vi "Infer top player action indicators.vi"(1 "Movement data with player transitions notated":string[][](array[string])=array1935x4[7740 elements]) -> (0 "Top player infered actions column":string[](array[string]))   [LabVIEW 2014]
panel:
  out "Top player action notated":string[][](array[string])
  out "Array 5":i32[][](array[numeric])
  out "Array":i32[][](array[numeric])
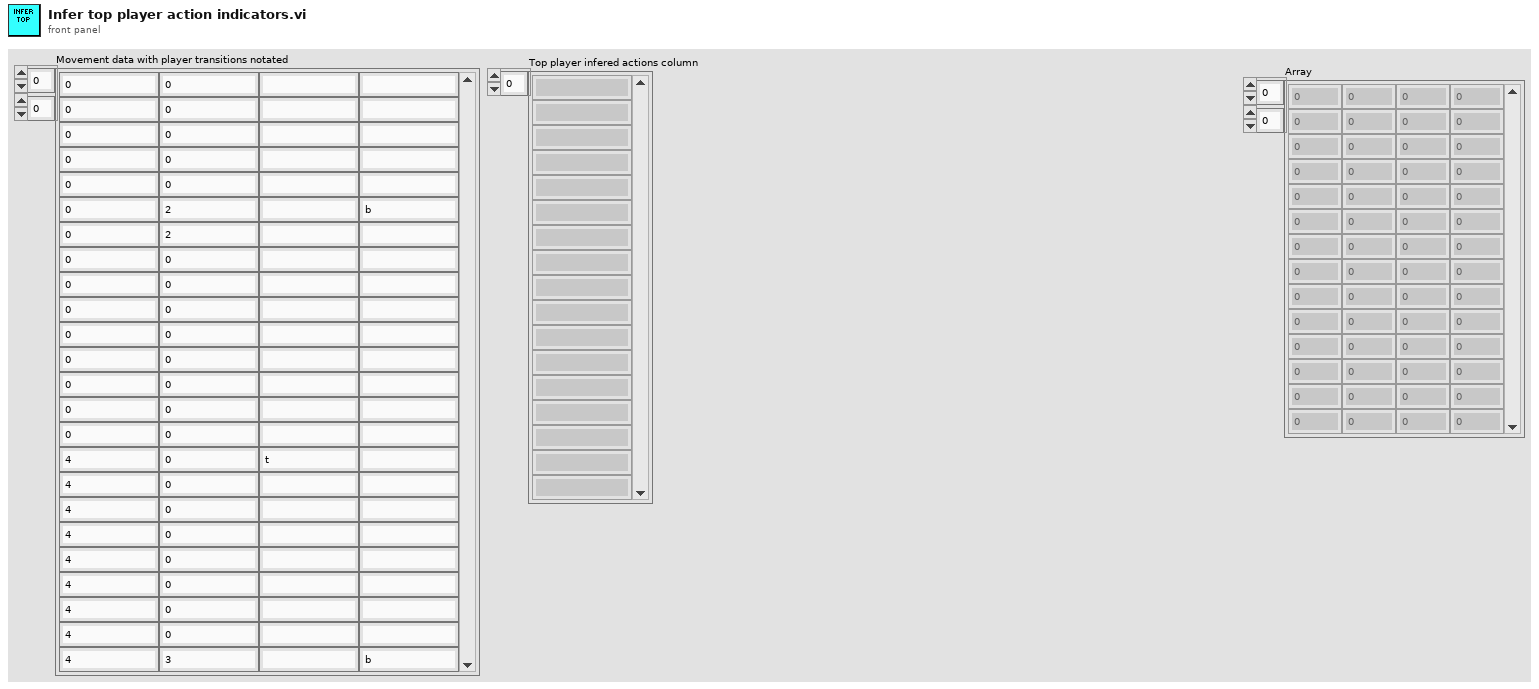
[diagram p1: front panel]
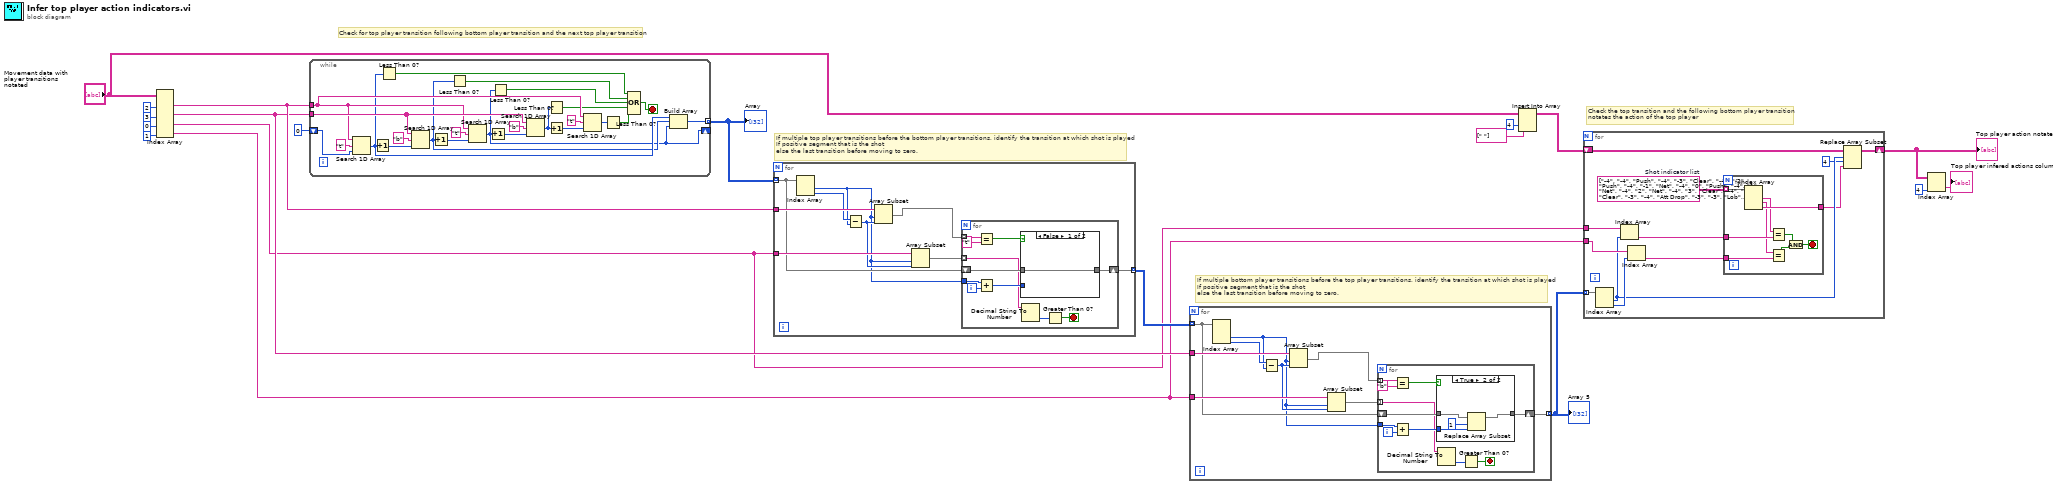
[diagram p0: block diagram]
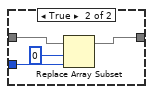
[diagram p3: hidden frame]
diagram:
  # "Check the top transition and the following bottom player transition\nnotates the action of the top player"
  # "If multiple bottom player transitions before the top player transitions, identify the transition at which shot is played\nIf positive segment that is the shot\nelse the last transition before moving to zero."
  # "If multiple top player transitions before the bottom player transitions, identify the transition at which shot is played\nIf positive segment that is the shot\nelse the last transition before moving to zero."
  # "Check for top player transition following bottom player transition and the next top player transition"
  n1 = Index Array(array="Movement data with player transitions notated", index (col) #1=2 ("disabled index (col)"), index (col) #2=3 ("index (col)"), index (col) #3=0 ("index (col)"), index (col) #4=1 ("index (col)")) -> (element #1=w16:string[], element #2=w12:string[], element #3=w8:string[], element #4=w9:string[])  [unwired: 4 in]
  n2 = while {
    tunnel: w16 -> [w33]
    tunnel: w12 -> [w34]
    shift-right: [w23] -> _
    shift-left: 0 ("index (col)") -> [w42]
    tunnel: [w39] -> w13 mode=indexing
    stop <- w26 stop-if-true
    n3 = Search 1D Array(1D array=w33, element="t", start index (0)=w42) -> (index of element=w25:i32)
    n4 = Increment(x=w25) -> (x+1=w38:i32)
    n5 = Less Than 0?(x=w25) -> (x < 0?=w22:bool)
    n6 = Search 1D Array(1D array=w34, element="b", start index (0)=w38) -> (index of element=w24:i32)
    n7 = Increment(x=w24) -> (x+1=w37:i32)
    n8 = Less Than 0?(x=w24) -> (x < 0?=w21:bool)
    n9 = Search 1D Array(1D array=w33, element="t", start index (0)=w37) -> (index of element=w23:i32)
    n10 = Increment(x=w23) -> (x+1=w35:i32)
    n11 = Less Than 0?(x=w23) -> (x < 0?=w20:bool)
    n12 = Search 1D Array(1D array=w34, element="b", start index (0)=w35) -> (index of element=w30:i32)
    n13 = Less Than 0?(x=w30) -> (x < 0?=w28:bool)
    n14 = Increment(x=w30) -> (x+1=w31:i32)
    n15 = Search 1D Array(1D array=w33, element="t", start index (0)=w31) -> (index of element=w29:i32)
    n16 = Less Than 0?(x=w29) -> (x < 0?=w27:bool)
    n17 = Compound Arithmetic op=OR(w22, w21, w20, w28, w27) -> (w26:bool)
    n18 = Build Array(w25, w24, w23) -> (w39:i32[])
  }
  "Array" <- w13
  n19 = for {
    tunnel: w13 -> [w46] mode=indexing
    tunnel: w16 -> [w52]
    tunnel: w8 -> [w50]
    tunnel: [w45] -> w11 mode=indexing
    n20 = Index Array(array=w46) -> (element #1=w44:i32, element #2=w51:i32)  [unwired: 2 in]
    n21 = Subtract(x=w51, y=w44) -> (x-y=w49:i32)
    n22 = Array Subset(array=w52, index=w44, length=w49) -> (w48:string[])
    n23 = Array Subset(array=w50, index=w44, length=w49) -> (w47:string[])
    n24 = for {
      tunnel: w48 -> [w63] mode=indexing
      tunnel: w47 -> [w56] mode=indexing
      tunnel: w44 -> [w60]
      shift-right: [w57] -> w45
      shift-left: w46 -> [w59]
      i -> [w61]
      stop <- w53 stop-if-true
      n25 = Equal?(x=w63, y="t") -> (x = y?=w55:bool)
      n26 = Add(x=w60, y=w61) -> (x+y=w58:i32)
      n27 = case shown="False" w55 {
        tunnel: w59 -> [w64 w68]
        tunnel: w58 -> [_ w67]
        tunnel: [w64 w65] -> w57
        frame False {
        }
        frame True {
          n28 = Replace Array Subset(array=w68, new element=w67, index=0) -> (w65:i32[])
        }
      }
      n29 = Decimal String To Number(string=w56) -> (number=w54:i32)  [unwired: 2 in, 1 out]
      n30 = Greater Than 0?(x=w54) -> (x > 0?=w53:bool)
    }
  }
  n31 = for {
    tunnel: w11 -> [w72] mode=indexing
    tunnel: w12 -> [w77]
    tunnel: w9 -> [w76]
    tunnel: [w71] -> w10 mode=indexing
    n32 = Index Array(array=w72) -> (element #2=w69:i32, element #3=w70:i32)  [unwired: 3 in, 1 out]
    n33 = Subtract(x=w70, y=w69) -> (x-y=w75:i32)
    n34 = Array Subset(array=w77, index=w69, length=w75) -> (w74:string[])
    n35 = Array Subset(array=w76, index=w69, length=w75) -> (w73:string[])
    n36 = for {
      tunnel: w74 -> [w88] mode=indexing
      tunnel: w73 -> [w81] mode=indexing
      tunnel: w69 -> [w85]
      shift-right: [w82] -> w71
      shift-left: w72 -> [w84]
      i -> [w86]
      stop <- w78 stop-if-true
      n37 = Equal?(x=w88, y="b") -> (x = y?=w80:bool)
      n38 = Add(x=w85, y=w86) -> (x+y=w83:i32)
      n39 = case shown="True" w80 {
        tunnel: w84 -> [w89 w93]
        tunnel: w83 -> [_ w92]
        tunnel: [w89 w90] -> w82
        frame False {
        }
        frame True {
          n40 = Replace Array Subset(array=w93, new element=w92, index=1) -> (w90:i32[])
        }
      }
      n41 = Decimal String To Number(string=w81) -> (number=w79:i32)  [unwired: 2 in, 1 out]
      n42 = Greater Than 0?(x=w79) -> (x > 0?=w78:bool)
    }
  }
  "Array 5" <- w10
  n43 = Insert Into Array(array="Movement data with player transitions notated", index (col)=4 ("disabled index (col)"), new element=string[] [" "] ("new element/subarray")) -> (w5:string[][])  [unwired: 1 in]
  n44 = for {
    tunnel: w10 -> [w105] mode=indexing
    tunnel: w9 -> [w103]
    tunnel: w8 -> [w104]
    shift-right: [w94] -> w3
    shift-left: w5 -> [w98]
    w101 = string[][] [["-4", "-4", "Push"], ["-4", "-3", "Clear"], ["-4", "-2", "Push"], ["-4", "-1", "Net"], ["-4", "0", "Push"], ["-4", "1", "Net"], ["-4", "2", "Net"], ["-4", "3", "Clear"], ["-4", "4", "Clear"], ["-3", "-4", "Att Drop"], ["-3", "-3", "Lob"], ["-3", "-2", "Att Drop"], ["-3", "-1", "Def Drop"], ["-3", "0", "Att Drop"], ["-3", "1", "Def Drop"], ["-3", "2", "Def Drop"], ["-3", "3", "Lob"], ["-3", "4", "Lob"], ["-2", "-4", "Push"], ["-2", "-3", "Clear"], ["-2", "-2", "Push"], ["-2", "-1", "Net"], ["-2", "0", "Push"], ["-2", "1", "Net"], ["-2", "2", "Net"], ["-2", "3", "Clear"], ["-2", "4", "Clear"], ["-1", "-4", "Deep Net"], ["-1", "-3", "Clear"], ["-1", "-2", "Deep Net"], ["-1", "-1", "Net"], ["-1", "0", "Deep Net"], ["-1", "1", "Net"], ["-1", "2", "Net"], ["-1", "3", "Clear"], ["-1", "4", "Clear"], ["0", "-4", "Push"], ["0", "-3", "Clear"], ["0", "-2", "Push"], ["0", "-1", "Net"], ["0", "0", "Push"], ["0", "1", "Net"], ["0", "2", "Net"], ["0", "3", "Clear"], ["0", "4", "Clear"], ["1", "-4", "Deep Net"], ["1", "-3", "Clear"], ["1", "-2", "Deep Net"], ["1", "-1", "Net"], ["1", "0", "Deep Net"], ["1", "1", "Net"], ["1", "2", "Net"], ["1", "3", "Clear"], ["1", "4", "Clear"], ["2", "-4", "Deep Net"], ["2", "-3", "Clear"], ["2", "-2", "Deep Net"], ["2", "-1", "Net"], ["2", "0", "Deep Net"], ["2", "1", "Net"], ["2", "2", "Net"], ["2", "3", "Clear"], ["2", "4", "Clear"], ["3", "-4", "Att Drop"], ["3", "-3", "Lob"], ["3", "-2", "Att Drop"], ["3", "-1", "Def Drop"], ["3", "0", "Att Drop"], ["3", "1", "Def Drop"], ["3", "2", "Def Drop"], ["3", "3", "Lob"], ["3", "4", "Lob"], ["4", "-4", "Att Drop"], ["4", "-3", "Lob"], ["4", "-2", "Att Drop"], ["4", "-1", "Def Drop"], ["4", "0", "Att Drop"], ["4", "1", "Def Drop"], ["4", "2", "Def Drop"], ["4", "3", "Lob"], ["4", "4", "Lob"]]  # Shot indicator list
    n45 = Index Array(array=w105) -> (element #1=w97:i32, element #2=w102:i32)  [unwired: 2 in]
    n46 = Index Array(array=w104, index=w97) -> (element=w100:string)
    n47 = Index Array(array=w103, index=w102) -> (element=w99:string)
    n48 = for {
      tunnel: w101 -> [w114] mode=indexing
      tunnel: [w113] -> w95
      tunnel: w100 -> [w112]
      tunnel: w99 -> [w110]
      stop <- w106 stop-if-true
      n49 = Index Array(array=w114) -> (element #1=w111:string, element #2=w109:string, element #3=w113:string)  [unwired: 3 in]
      n50 = Equal?(x=w111, y=w112) -> (x = y?=w108:bool)
      n51 = Equal?(x=w109, y=w110) -> (x = y?=w107:bool)
      n52 = And(x=w108, y=w107) -> (x .and. y?=w106:bool)
    }
    n53 = Replace Array Subset(array=w98, new element=w95, index (row)=w97, index (col)=4 ("disabled index (col)")) -> (w94:string[][])
  }
  "Top player action notated" <- w3
  n54 = Index Array(array=w3, index (col)=4 ("disabled index (col)")) -> (element=→"Top player infered actions column":string[])  [unwired: 1 in]
